vi "MHTML Header.vi"() -> (2 "MHTML Header":string, 3 "boundary":string)   [LabVIEW 2011]
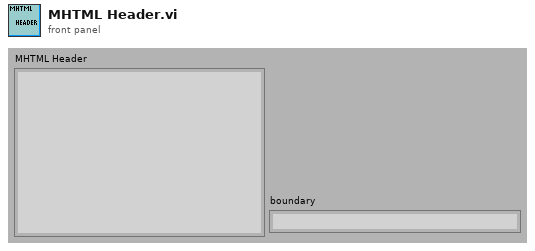
[diagram p1: front panel]
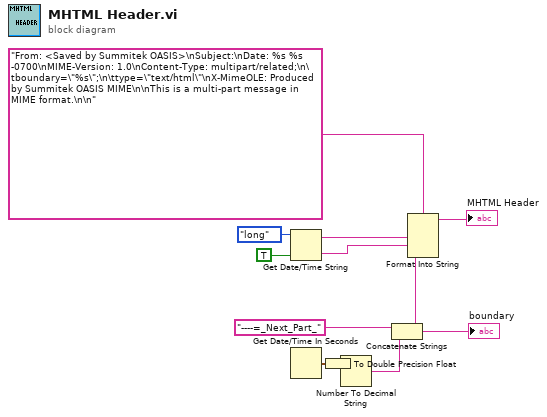
[diagram p0: block diagram]
diagram:
  n1 = Get Date/Time String(date format (0)=enum16{"short", "long", "abbreviated"}."long", want seconds? (F)=TRUE) -> (date string=w7:string, time string=w6:string)  [unwired: 1 out]
  n2 = Get Date/Time In Seconds() -> (seconds since 1Jan1904=w1:timestamp)
  n3 = To Double Precision Float(number=w1) -> (double precision float=w9:dbl)
  n4 = Number To Decimal String(number=w9) -> (decimal integer string=w3:string)  [unwired: 1 out]
  n5 = Concatenate Strings("----=_Next_Part_", w3) -> (w2:string)
  "boundary" <- w2
  n6 = Format Into String(format string="From: <Saved by Summitek OASIS>\nSubject:\nDate: %s %s -0700\nMIME-Version: 1.0\nContent-Type: multipart/related;\n\tboundary=\"%s\";\n\ttype=\"text/html\"\nX-MimeOLE: Produced by Summitek OASIS MIME\n\nThis is a multi-part message in MIME format.\n\n", w7, w6, w2) -> (resulting string=→"MHTML Header":string)  [unwired: 2 in, 1 out]
